vi "Read Msg.vi"(7 "Actor in":refnum<class "Actor.lvclass">) -> (2 "Msg":refnum<class "Msg.lvclass">)   [LabVIEW 2020, in "jettl.lvlib" / "Actor Specific.lvlib"]
uses:
  Actor Specific.lvlib
  Actor/Actor.lvclass
  Msg/Msg.lvclass
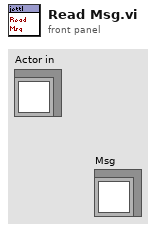
[diagram p1: front panel]
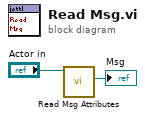
[diagram p0: block diagram]
diagram:
  n1 = call-dynamic "Read Msg Attributes.vi"("Actor in"="Actor in") -> ("Msg"=→"Msg":refnum<class "Msg.lvclass">)  [unwired: 10 in]
